vi "Eval Formula Node.vi"(0 "Variables Input":string[](array[string]), 1 "Input Values":dbl[](array[numeric]), 2 "Variables Output":string[](array[string]), 3 "formula":string, 4 "error in (no error)":errorcluster) -> (5 "Output Values":dbl[](array[numeric]), 6 "error out":errorcluster)   [LabVIEW 2017, in "NI_Gmath.lvlib"]
doc: "Similar to the Formula Node but with variables that can be entered on the front panel. Refer to Formula Parsing VIs in More Detail for more information on the differences between the Eval Formula Node VI and the Formula Node."
uses:
  NI_Gmath.lvlib
panel:
  # "Example:\n\n Variables Input: a and b\n Input Values: 1.0 and 2.0 \n Variables Output: x and y \n formula: x=a+b; y=a*b;"
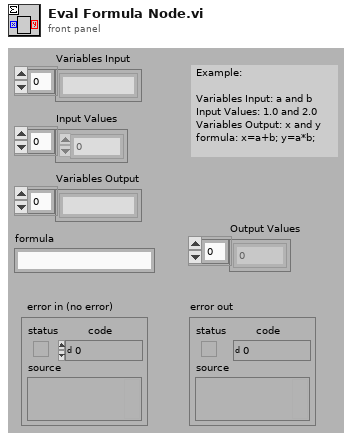
[diagram p1: front panel]
types:
  T1 = cluster{"Y Values":dbl[][], "Tables":i32[][][], "Variables input decode":i32[], "Variables output decode":i32[]}
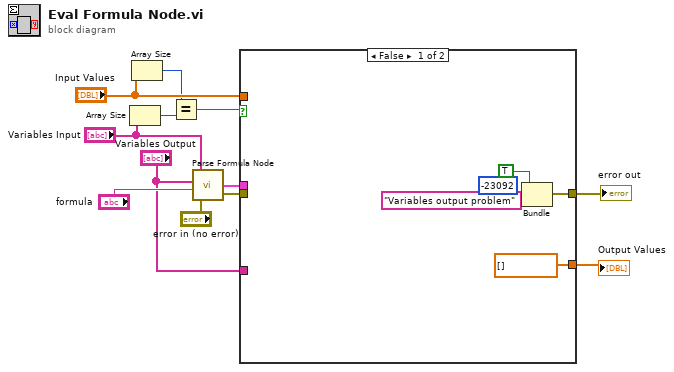
[diagram p0: block diagram]
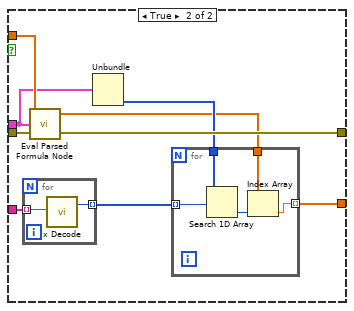
[diagram p2: hidden frame]
diagram:
  n1 = Array Size(array="Variables Input") -> (size(s)=w4:i32)
  n2 = Array Size(array="Input Values") -> (size(s)=w5:i32)
  n3 = Equal?(x=w5, y=w4) -> (x = y?=w3:bool)
  n4 = call "Parse Formula Node.vi"("error in (no error)"="error in (no error)", "formula"="formula", "Variables Output"="Variables Output", "Variables Input"="Variables Input") -> ("error out"=w9:errorcluster, "Parsed Formula Node"=w8:T1)
  n5 = case shown="False" w3 {
    tunnel: "Input Values" -> [_ w26]
    tunnel: w8 -> [_ w25]
    tunnel: w9 -> [_ w24]
    tunnel: [w14 w23] -> w12
    tunnel: "Variables Output" -> [_ w22]
    tunnel: [dbl[] [] ("Output Values") w18] -> w1
    frame False {
      n6 = Bundle(TRUE, -23092, "Variables output problem") -> (w14:errorcluster)  [unwired: 1 in]
    }
    frame True {
      n7 = for {
        tunnel: w22 -> [w33] mode=indexing
        tunnel: [w32] -> w20 mode=indexing
        n8 = call "x Decode.vi"("x string"=w33) -> ("number"=w32:i32)  [unwired: 1 in, 1 out]
      }
      n9 = call "Eval Parsed Formula Node.vi"("error in (no error)"=w24, "Parsed Formula Node"=w25, "Input Values"=w26) -> ("error out"=w23:errorcluster, "Output Values"=w19:dbl[])
      n10 = Unbundle(w25) -> ("Variables output decode"=w21:i32[])  [unwired: 3 out]
      n11 = for {
        tunnel: w21 -> [w31]
        tunnel: w20 -> [w30] mode=indexing
        tunnel: w19 -> [w28]
        tunnel: [w27] -> w18 mode=indexing
        n12 = Search 1D Array(1D array=w31, element=w30) -> (index of element=w29:i32)  [unwired: 1 in]
        n13 = Index Array(array=w28, index=w29) -> (element=w27:dbl)
      }
    }
  }
  "Output Values" <- w1
  "error out" <- w12
